vi "dui.vi"() -> ()   [LabVIEW 2014]
doc: "该模板用于创建生产者／消费者模式的应用程序。该模板可用于执行诸如数据分析的数据处理，或者在以不均匀速率产生数据的数据源中（如触发采集），当数据可用时对数据进行分析。"
uses:
  <vilib>/vision/Image Controls.llb/IMAQ Image.ctl
panel:
  out "毫秒计时值":u32
  out "Image Pixels (U8)":u8[][](array[numeric])
  in  "stop":bool caption="停止"
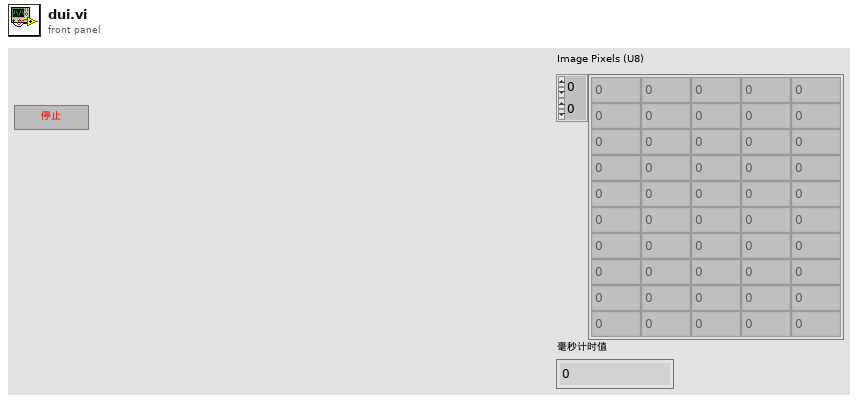
[diagram p1: front panel]
types:
  T1 = typedef "IMAQ Image.ctl" = refnum<image>
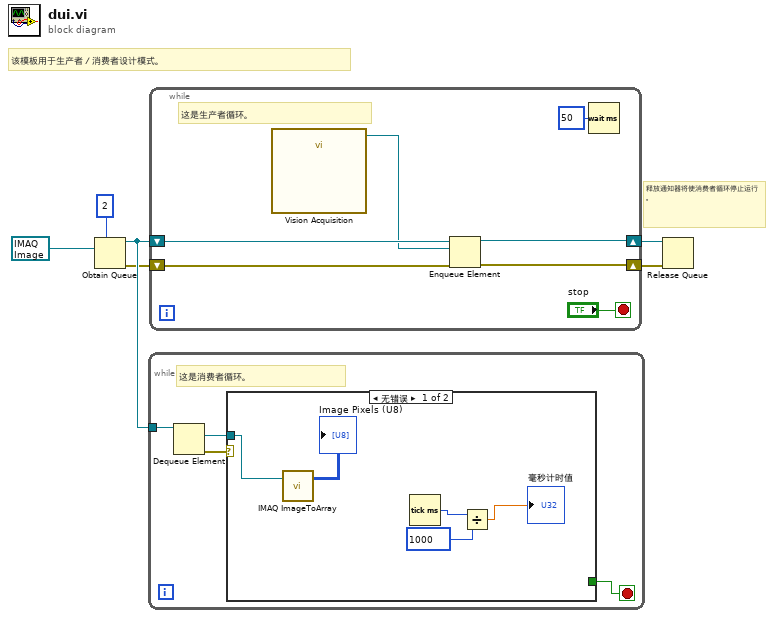
[diagram p0: block diagram]
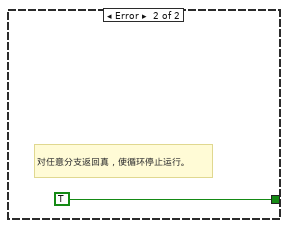
[diagram p2: hidden frame]
diagram:
  # "释放通知器将使消费者循环停止运行。"
  # "该模板用于生产者／消费者设计模式。"
  n1 = Obtain Queue(max queue size (-1, unlimited)=2 ("队列最大值（-1，无限）"), element data type=T1 refnum ("Image Out")) -> (queue out=w6:refnum<queue>, error out=w5:errorcluster)  [unwired: 3 in, 1 out]
  n2 = while {
    tunnel: w6 -> [w10]
    stop <- w7 stop-if-true
    # "这是消费者循环。"
    n3 = Dequeue Element(queue=w10) -> (element=w8:T1, error out=w9:errorcluster)  [unwired: 2 in, 2 out]
    n4 = case shown="无错误" w9 {
      tunnel: w8 -> [w15 _]
      tunnel: [_ TRUE] -> w7
      frame No Error {
        n5 = call "IMAQ ImageToArray"("Image"=w15) -> ("Image Pixels (U8)"=→"Image Pixels (U8)":u8[][])  [unwired: 3 in, 4 out]
        n6 = Tick Count (ms)() -> (millisecond timer value=w13:u32)
        n7 = Divide(x=w13, y=u32 1000) -> (x/y=→"毫秒计时值":dbl)
      }
      frame Error {
        # "对任意分支返回真，使循环停止运行。"
      }
    }
  }
  n8 = while {
    shift-right: [w19] -> w3
    shift-left: w5 -> [w20]
    shift-right: [w21] -> w4
    shift-left: w6 -> [w22]
    stop <- "stop" stop-if-true
    # "这是生产者循环。"
    n9 = call "Vision Acquisition"() -> ("Image Out"=w17:T1)  [unwired: 26 in, 1 out]
    n10 = Enqueue Element(queue=w22, element=w17, error in (no error)=w20) -> (queue out=w21:refnum<queue>, error out=w19:errorcluster)  [unwired: 1 in, 1 out]
    n11 = Wait (ms)(milliseconds to wait=u32 50) -> ()  [unwired: 1 out]
  }
  n12 = Release Queue(queue=w4, error in (no error)=w3) -> ()  [unwired: 1 in, 3 out]
